vi "c_DECLARE_IO.vi"(11 "TopLevelDiagram in":refnum<vi>) -> (3 "CodeElements":refnum<class "CodeElement.lvclass">[](array[class]))   [LabVIEW 2017]
uses:
  CodeElements/Base/CodeElement.lvclass
  CodeElements/Typedef_Element_class/Typedef_Element.lvclass
  E:/Code_Generator/CodeElements/Base/CodeElement.lvclass
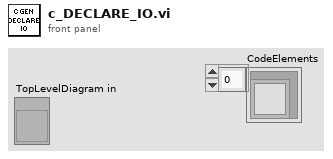
[diagram p1: front panel]
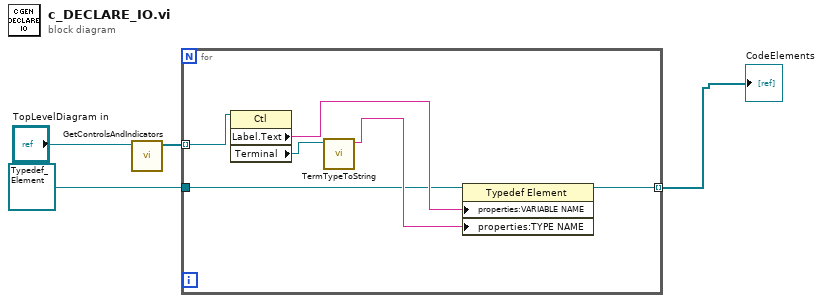
[diagram p0: block diagram]
diagram:
  n1 = call "GetControlsAndIndicators.vi"("TopLevelDiagram in"="TopLevelDiagram in") -> ("All ControlsTerminals"=w4:refnum<vi>[])  [unwired: 9 in, 1 out]
  n2 = for {
    tunnel: w4 -> [w10] mode=indexing
    tunnel: refnum<class "Typedef_Element.lvclass"> refnum ("Variable_Declaration") -> [w5]
    tunnel: [w6] -> w1 mode=indexing
    n3 = property class="Ctl"(reference=w10) -> ("Label.Text"=w8:string, "Terminal"=w9:refnum<vi>)  [unwired: 1 in, 2 out]
    n4 = call "TermTypeToString.vi"("Terminal in"=w9) -> ("Name"=w7:string)  [unwired: 10 in]
    n5 = property class="Typedef Element"(reference=w5, "properties:VARIABLE NAME"=w8, "properties:TYPE NAME"=w7) -> (reference out=w6:refnum<class "Typedef_Element.lvclass">)  [unwired: 1 in, 1 out]
  }
  "CodeElements" <- w1
